vi "参数设置1.1.vi"(0 "X轴速度":dbl=9000.0, 1 "精度":dbl=0.001, 2 "细分设置":dbl=8.0, 3 "等待时间":dbl=40.0, 5 "X轴回零速度":dbl=15000.0, 9 "Y轴速度":dbl=9000.0, 11 "Y轴回零速度":dbl=15000.0) -> (4 "X轴速度":dbl=9000.0, 6 "X轴回零速度":dbl=15000.0, 8 "采样阶":dbl=11.0, 10 "Y轴速度":dbl=9000.0, 12 "精度":dbl=0.001, 13 "细分设置":dbl=8.0, 14 "等待时间":dbl=40.0, 15 "Y轴回零速度":dbl=15000.0)   [LabVIEW 2016]
panel:
  in  "确定":bool
  in  "选项卡控件":enum32{"控制参数", "X轴", "Y轴", "采集卡"}(tab)=enum."采集卡"
  in  "采样数阶":dbl=12.0
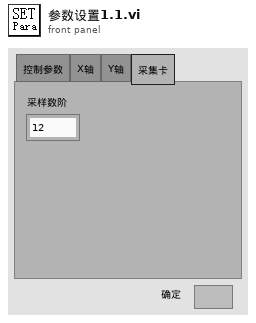
[diagram p1: front panel]
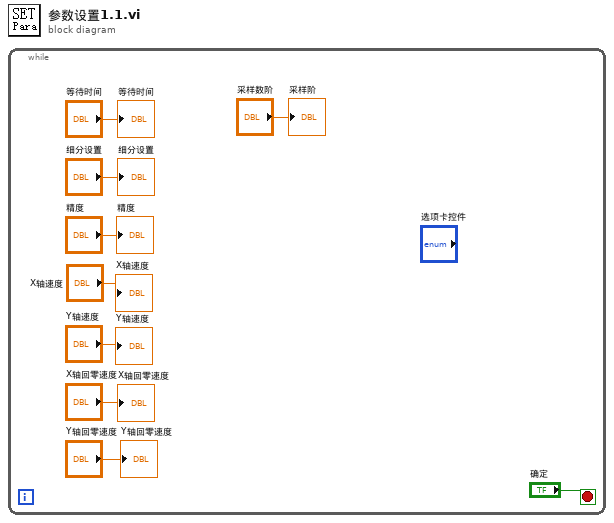
[diagram p0: block diagram]
diagram:
  n1 = while {
    stop <- "确定" stop-if-true
    "等待时间" <- "等待时间"
    "细分设置" <- "细分设置"
    "精度" <- "精度"
    "X轴速度" <- "X轴速度"
    "Y轴速度" <- "Y轴速度"
    "X轴回零速度" <- "X轴回零速度"
    "Y轴回零速度" <- "Y轴回零速度"
    "采样阶" <- "采样数阶"
  }
